vi "File_save(SubVI).vi"(8 "Numeric":dbl, 9 "Array":dbl[](array[numeric]), 10 "Save to file":bool, 11 "file path (dialog if empty)":path) -> ()   [LabVIEW 2017]
doc: "SubVi that save data from <B>Array</B> into file when <B>Save to File</B> is true and <B>Numeric</B> is equal to 4"
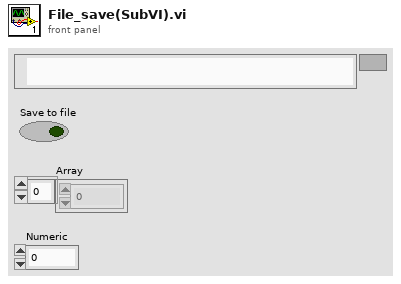
[diagram p1: front panel]
types:
  T1 = enum16{"open", "replace", "create", "open or create", "replace or create", "replace or create with confirmation"}
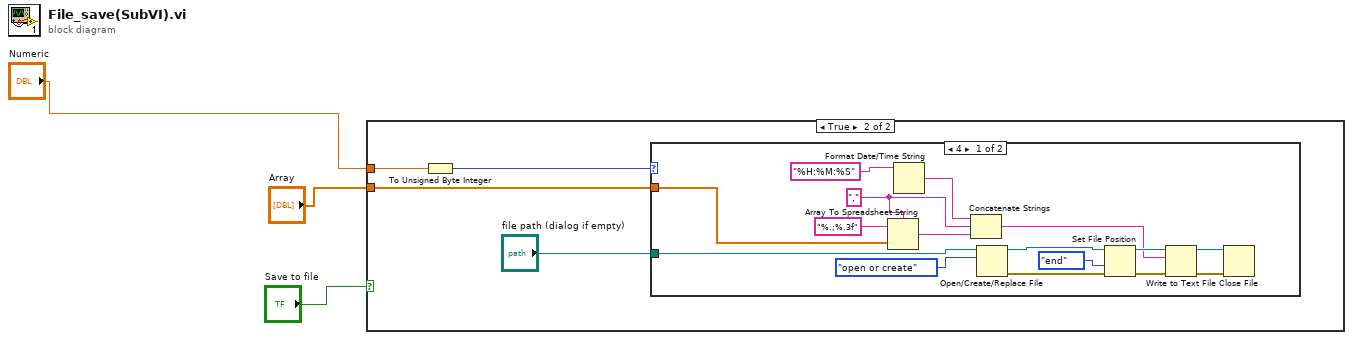
[diagram p0: block diagram]
diagram:
  n1 = case shown="True" "Save to file" {
    tunnel: "Numeric" -> [_ w5]
    tunnel: "Array" -> [_ w7]
    frame False {
    }
    frame True {
      n2 = To Unsigned Byte Integer(number=w5) -> (unsigned 8bit integer=w4:u8)
      n3 = case shown="4" w4 {
        tunnel: w7 -> [w22 _]
        tunnel: "file path (dialog if empty)" -> [w11 _]
        frame 4 {
          w12 = "," ("delimiter (Tab)")
          n4 = Array To Spreadsheet String(delimiter (Tab)=w12, array=w22, 3:"%.;%.3f" ("format string")) -> (spreadsheet string=w20:string)
          n5 = Format Date/Time String(time format string (%c)="%H:%M:%S") -> (date/time string=w21:string)  [unwired: 2 in]
          n6 = Concatenate Strings(w21, w12, w20) -> (w16:string)
          n7 = Open/Create/Replace File(file path (use dialog)=w11, operation (0:open)=T1."open or create") -> (refnum out=w10:refnum<file>, error out=w9:errorcluster)  [unwired: 4 in, 1 out]
          n8 = Set File Position(refnum=w10, from (0:start)=enum16{"start", "end", "current"}."end", error in=w9) -> (refnum out=w18:refnum<file>, error out=w17:errorcluster)  [unwired: 1 in]
          n9 = Write to Text File(file (use dialog)=w18, text=w16, error in=w17) -> (refnum out=w15:refnum<file>, error out=w14:errorcluster)  [unwired: 1 in, 1 out]
          n10 = Close File(refnum=w15, error in=w14) -> ()  [unwired: 2 out]
        }
        frame Default {
        }
      }
    }
  }
